vi "Range Index.vi"(1 "Index":i32, 2 "Size":i32) -> (3 "Index Out Out":i32)   [LabVIEW 2020, in "Index_Pointer.lvclass"]
uses:
  Index_Pointer.lvclass
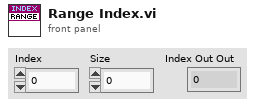
[diagram p1: front panel]
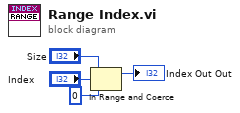
[diagram p0: block diagram]
diagram:
  n1 = In Range and Coerce(upper limit="Size", x="Index", lower limit=0) -> (coerced(x)=→"Index Out Out":i32)  [unwired: 1 out]
